vi "DeleteFakeStatusFrom_DotMatrix1.vi"(2 "error IN":errorcluster, 3 "Source Matrix":i16[][](array[numeric])) -> (0 "error OUT":errorcluster, 1 "Filtered Dot Matrix":i16[][](array[numeric]))   [LabVIEW 2013]
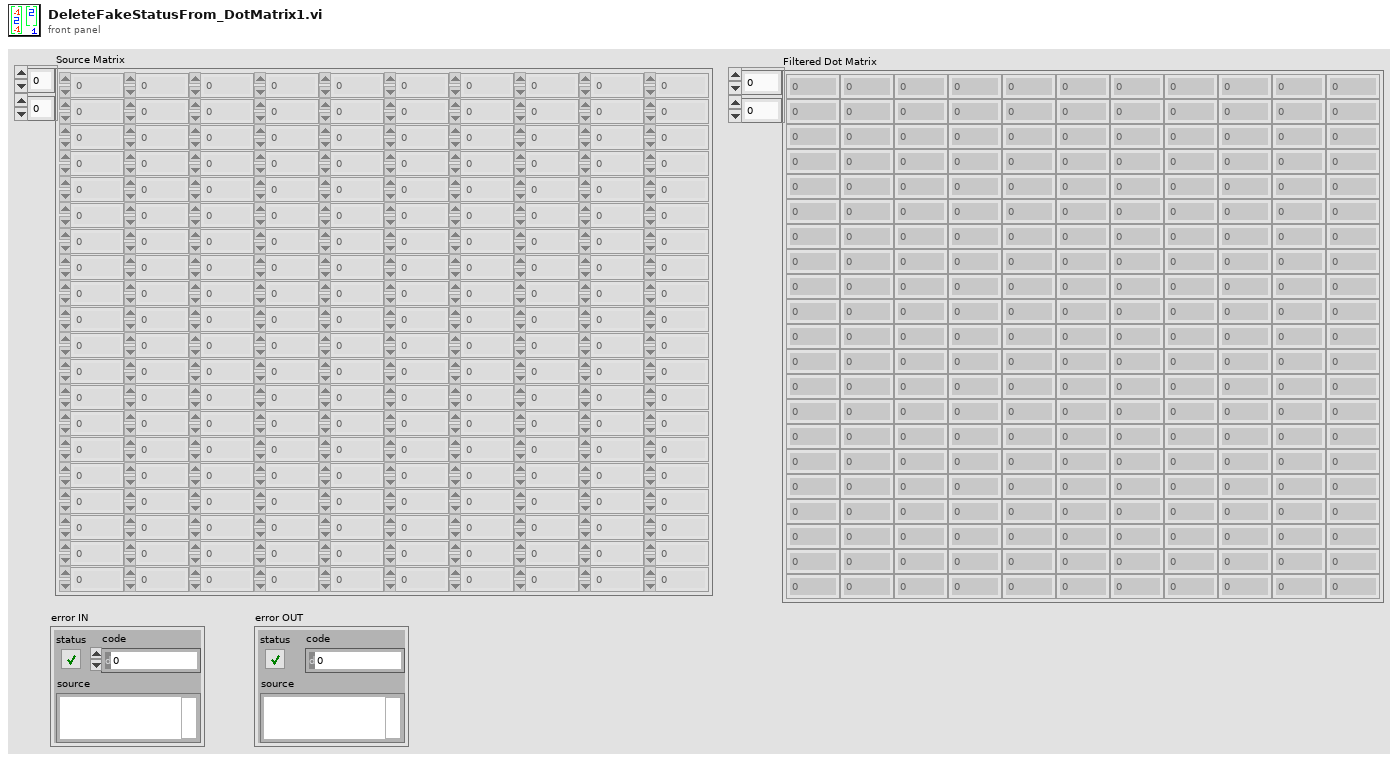
[diagram p1: front panel]
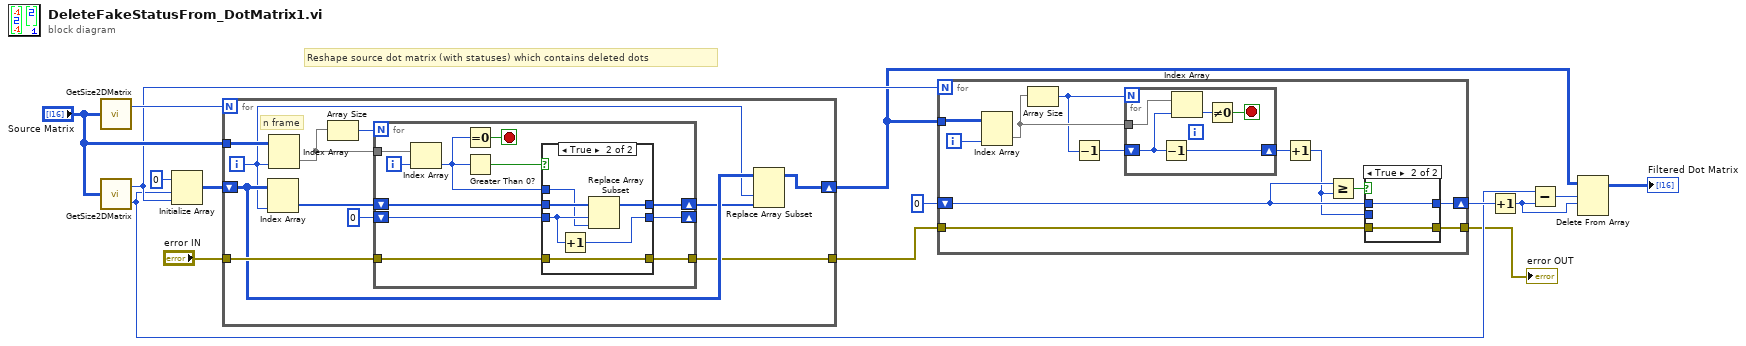
[diagram p0: block diagram]
diagram:
  # "Reshape source dot matrix (with statuses) which contains deleted dots"
  n1 = call "GetSize2DMatrix.vi"("Array IN (2D)"="Source Matrix") -> ("# Cols"=w11:i32)  [unwired: 1 out]
  n2 = call "GetSize2DMatrix.vi"("Array IN (2D)"="Source Matrix") -> ("# Cols"=w6:i32, "# Rows"=w5:i32)
  n3 = Initialize Array(i16 0 ("element"), w5, w6) -> (w13:i16[][])
  n4 = for {
    N: w11 -> [_]
    tunnel: "Source Matrix" -> [w26]
    shift-right: [w22] -> w2
    shift-left: w13 -> [w23]
    tunnel: "error IN" -> [w24]
    tunnel: [w19] -> w4
    i -> [w21]
    # "n frame"
    n5 = Index Array(array=w23, index (col)=w21) -> (element=w18:i16[])  [unwired: 1 in]
    n6 = Index Array(array=w26, index (col)=w21) -> (element=w17:i16[])  [unwired: 1 in]
    n7 = Array Size(array=w17) -> (size(s)=w16:i32)
    n8 = for {
      N: w16 -> [_]
      tunnel: w17 -> [w31]
      shift-right: [w34] -> w20
      shift-left: w18 -> [w37]
      shift-right: [w35] -> _
      shift-left: 0 -> [w36]
      tunnel: w24 -> [w33]
      tunnel: [w32] -> w19
      i -> [w30]
      stop <- w29 stop-if-true
      n9 = Index Array(array=w31, index=w30) -> (element=w27:i16)
      n10 = Equal To 0?(x=w27) -> (x = 0?=w29:bool)
      n11 = Greater Than 0?(x=w27) -> (x > 0?=w28:bool)
      n12 = case shown="True" w28 {
        tunnel: w37 -> [w40 w46]
        tunnel: w36 -> [w39 w45]
        tunnel: [w39 w43] -> w35
        tunnel: [w40 w42] -> w34
        tunnel: w33 -> [w38 w44]
        tunnel: [w38 w44] -> w32
        tunnel: w27 -> [_ w41]
        frame False {
        }
        frame True {
          n13 = Increment(x=w45) -> (x+1=w43:i32)
          n14 = Replace Array Subset(array=w46, new element=w41, index=w45) -> (w42:i16[])
        }
      }
    }
    n15 = Replace Array Subset(array=w23, new element=w20, index (col)=w21) -> (w22:i16[][])  [unwired: 1 in]
  }
  n16 = for {
    N: w6 -> [_]
    tunnel: w2 -> [w58]
    shift-right: [w53] -> w7
    shift-left: 0 -> [w54]
    tunnel: w4 -> [w48]
    tunnel: [w47] -> w3
    i -> [w57]
    n17 = Index Array(array=w58, index (col)=w57) -> (element=w56:i16[])  [unwired: 1 in]
    n18 = Array Size(array=w56) -> (size(s)=w49:i32)
    n19 = Decrement(x=w49) -> (x-1=w52:i32)
    n20 = for {
      N: w49 -> [_]
      tunnel: w56 -> [w67]
      shift-right: [w65] -> w51
      shift-left: w52 -> [w63]
      stop <- w64 stop-if-true
      n21 = Decrement(x=w63) -> (x-1=w65:i32)
      n22 = Index Array(array=w67, index=w63) -> (element=w66:i16)
      n23 = Not Equal To 0?(x=w66) -> (x != 0?=w64:bool)
    }
    n24 = Increment(x=w51) -> (x+1=w50:i32)
    n25 = Greater Or Equal?(x=w54, y=w50) -> (x >= y?=w55:bool)
    n26 = case shown="True" w55 {
      tunnel: w54 -> [_ w62]
      tunnel: [w60 w62] -> w53
      tunnel: w50 -> [w60 _]
      tunnel: w48 -> [w59 w61]
      tunnel: [w59 w61] -> w47
      frame False {
      }
      frame True {
      }
    }
  }
  "error OUT" <- w3
  n27 = Increment(x=w7) -> (x+1=w8:i32)
  n28 = Subtract(x=w5, y=w8) -> (x-y=w9:i32)
  n29 = Delete From Array(array=w2, length=w9, index (row)=w8) -> (array with subset deleted=→"Filtered Dot Matrix":i16[][])  [unwired: 1 in, 1 out]
